vi "Set All Session Data.vi"(7 "Database Connection":refnum<k7>, 8 "Error In":errorcluster) -> (0 "Error Out":errorcluster)   [LabVIEW 2019]
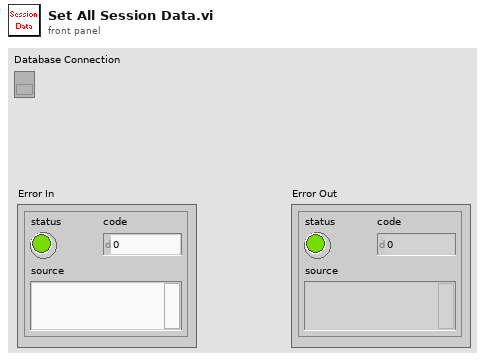
[diagram p1: front panel]
types:
  T1 = typedef "Device Settings.ctl" = cluster{"Device Type":string, "Device Name":string, "DAQmx Name":tag, "Terminal Wiring":i32}
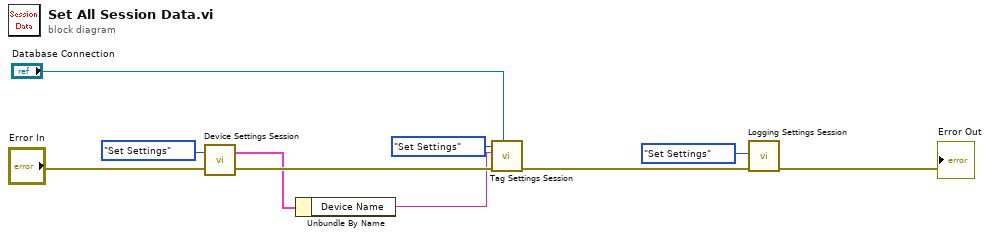
[diagram p0: block diagram]
diagram:
  n1 = call "Device Settings Session.vi"("Error In"="Error In", "Type"=enum16{"Set Settings", "Get Settings"}."Set Settings") -> ("Error Out"=w6:errorcluster, "Device Settings"=w2:T1)
  n2 = Unbundle By Name(w2) -> ("Device Name"=w1:string)
  n3 = call "Tag Settings Session.vi"("Database Connection"="Database Connection", "Error In"=w6, "DeviceName"=w1, "Type"=enum16{"Set Settings", "Get Settings"}."Set Settings") -> ("Error Out"=w5:errorcluster)  [unwired: 6 in, 1 out]
  n4 = call "Logging Settings Session.vi"("Type"=enum16{"Set Settings", "Get Settings"}."Set Settings", "Error In"=w5) -> ("Error Out"=→"Error Out":errorcluster)  [unwired: 12 in, 1 out]
